vi "DevScripts_EnumToEnumAndLookup.vi"() -> ()   [LabVIEW 2024]
uses:
  <vilib>/regexp/Match Regular Expression.xnode
  SDL3/Pixels/PixelFormat--enum.ctl
  SDL3/Pixels/Pixels.lvlib
panel:
  out "Array":string[](array[string])
  out "Lookup":u32[](array[numeric]) format="%.0x"
  in  "#Define list":string="SDL_PIXELFORMAT_UNKNOWN = 0,\n    SDL_PIXELFORMAT_INDEX1LSB = 0x11100100u,\n        /* SDL_DEFINE_PIXELFORMAT(SDL_PIXELTYPE_INDEX1, SDL_BITMAPORDER_4321, 0, 1, 0), */\n    SDL_PIXELFORMAT_INDEX1MSB = 0x11200100u,\n        /* SDL_DEFINE_PIXELFORMAT(SDL_PIXELTYPE_INDEX1, SDL_BITMAPORDER_1234, 0, 1, 0), */\n    SDL_PIXELFORMAT_INDEX2LSB = 0x1c100200u,\n        /* SDL_DEFINE_PIXELFORMAT(SDL_PIXELTYPE_INDEX2, SDL_BITMAPORDER_4321, 0, 2, 0), */\n    SDL_PIXELFORMAT_INDEX2MSB = 0x1c200200u,\n        /* SDL_DEFINE_PIXELFORMAT(SDL_PIXELTYPE_INDEX2, SDL_BITMAPORDER_1234, 0, 2, 0), */\n    SDL_PIXELFORMAT_INDEX4LSB = 0x12100400u,\n        /* SDL_DEFINE_PIXELFORMAT(SDL_PIXELTYPE_INDEX4, SDL_BITMAPORDER_4321, 0, 4, 0), */\n    SDL_PIXELFORMAT_INDEX4MSB = 0x12200400u,\n        /* SDL_DEFINE_PIXELFORMAT(SDL_PIXELTYPE_INDEX4, SDL_BITMAPORDER_1234, 0, 4, 0), */\n    SDL_PIXELFORMAT_INDEX8 = 0x13000801u,\n        /* SDL_DEFINE_PIXELFORMAT(SDL_PIXELTYPE_INDEX8, 0, 0, 8, 1), */\n    SDL_PIXELFORMAT_RGB332 = 0x14110801u,\n        /* SDL_DEFINE_PIXELFORMAT(SDL_PIXELTYPE_PACKED8, SDL_PACKEDORDER_XRGB, SDL_PACKEDLAYOUT_332, 8, 1), */\n    SDL_PIXELFORMAT_XRGB4444 = 0x15120c02u,\n        /* SDL_DEFINE_PIXELFORMAT(SDL_PIXELTYPE_PACKED16, SDL_PACKEDORDER_XRGB, SDL_PACKEDLAYOUT_4444, 12, 2), */\n    SDL_PIXELFORMAT_XBGR4444 = 0x15520c02u,\n        /* SDL_DEFINE_PIXELFORMAT(SDL_PIXELTYPE_PACKED16, SDL_PACKEDORDER_XBGR, SDL_PACKEDLAYOUT_4444, 12, 2), */\n    SDL_PIXELFORMAT_XRGB1555 = 0x15130f02u,\n        /* SDL_DEFINE_PIXELFORMAT(SDL_PIXELTYPE_PACKED16, SDL_PACKEDORDER_XRGB, SDL_PACKEDLAYOUT_1555, 15, 2), */\n    SDL_PIXELFORMAT_XBGR1555 = 0x15530f02u,\n        /* SDL_DEFINE_PIXELFORMAT(SDL_PIXELTYPE_PACKED16, SDL_PACKEDORDER_XBGR, SDL_PACKEDLAYOUT_1555, 15, 2), */\n    SDL_PIXELFORMAT_ARGB4444 = 0x15321002u,\n        /* SDL_DEFINE_PIXELFORMAT(SDL_PIXELTYPE_PACKED16, SDL_PACKEDORDER_ARGB, SDL_PACKEDLAYOUT_4444, 16, 2), */\n    SDL_PIXELFORMAT_RGBA4444 = 0x15421002u,\n        /* SDL_DEFINE_PIXELFORMAT(SDL_PIXELTYPE_PACKED16, SDL_PACKEDORDER_RGBA, SDL_PACKEDLAYOUT_4444, 16, 2), */\n    SDL_PIXELFORMAT_ABGR4444 = 0x15721002u,\n        /* SDL_DEFINE_PIXELFORMAT(SDL_PIXELTYPE_PACKED16, SDL_PACKEDORDER_ABGR, SDL_PACKEDLAYOUT_4444, 16, 2), */\n    SDL_PIXELFORMAT_BGRA4444 = 0x15821002u,\n        /* SDL_DEFINE_PIXELFORMAT(SDL_PIXELTYPE_PACKED16, SDL_PACKEDORDER_BGRA, SDL_PACKEDLAYOUT_4444, 16, 2), */\n    SDL_PIXELFORMAT_ARGB1555 = 0x15331002u,\n        /* SDL_DEFINE_PIXELFORMAT(SDL_PIXELTYPE_PACKED16, SDL_PACKEDORDER_ARGB, SDL_PACKEDLAYOUT_1555, 16, 2), */\n    SDL_PIXELFORMAT_RGBA5551 = 0x15441002u,\n        /* SDL_DEFINE_PIXELFORMAT(SDL_PIXELTYPE_PACKED16, SDL_PACKEDORDER_RGBA, SDL_PACKEDLAYOUT_5551, 16, 2), */\n    SDL_PIXELFORMAT_ABGR1555 = 0x15731002u,\n        /* SDL_DEFINE_PIXELFORMAT(SDL_PIXELTYPE_PACKED16, SDL_PACKEDORDER_ABGR, SDL_PACKEDLAYOUT_1555, 16, 2), */\n    SDL_PIXELFORMAT_BGRA5551 = 0x15841002u,\n        /* SDL_DEFINE_PIXELFORMAT(SDL_PIXELTYPE_PACKED16, SDL_PACKEDORDER_BGRA, SDL_PACKEDLAYOUT_5551, 16, 2), */\n    SDL_PIXELFORMAT_RGB565 = 0x15151002u,\n        /* SDL_DEFINE_PIXELFORMAT(SDL_PIXELTYPE_PACKED16, SDL_PACKEDORDER_XRGB, SDL_PACKEDLAYOUT_565, 16, 2), */\n    SDL_PIXELFORMAT_BGR565 = 0x15551002u,\n        /* SDL_DEFINE_PIXELFORMAT(SDL_PIXELTYPE_PACKED16, SDL_PACKEDORDER_XBGR, SDL_PACKEDLAYOUT_565, 16, 2), */\n    SDL_PIXELFORMAT_RGB24 = 0x17101803u,\n        /* SDL_DEFINE_PIXELFORMAT(SDL_PIXELTYPE_ARRAYU8, SDL_ARRAYORDER_RGB, 0, 24, 3), */\n    SDL_PIXELFORMAT_BGR24 = 0x17401803u,\n        /* SDL_DEFINE_PIXELFORMAT(SDL_PIXELTYPE_ARRAYU8, SDL_ARRAYORDER_BGR, 0, 24, 3), */\n    SDL_PIXELFORMAT_XRGB8888 = 0x16161804u,\n        /* SDL_DEFINE_PIXELFORMAT(SDL_PIXELTYPE_PACKED32, SDL_PACKEDORDER_XRGB, SDL_PACKEDLAYOUT_8888, 24, 4), */\n    SDL_PIXELFORMAT_RGBX8888 = 0x16261804u,\n        /* SDL_DEFINE_PIXELFORMAT(SDL_PIXELTYPE_PACKED32, SDL_PACKEDORDER_RGBX, SDL_PACKEDLAYOUT_8888, 24, 4), */\n    SDL_PIXELFORMAT_XBGR8888 = 0x16561804u,\n        /* SDL_DEFINE_PIXELFORMAT(SDL_PIXELTYPE_PACKED32, SDL_PACKEDORDER_XBGR, SDL_PACKEDLAYOUT_8888, 24, 4), */\n    SDL_PIXELFORMAT_BGRX8888 = 0x16661804u,\n        /* SDL_DEFINE_PIXELFORMAT(SDL_PIXELTYPE_PACKED32, SDL_PACKEDORDER_BGRX, SDL_PACKEDLAYOUT_8888, 24, 4), */\n    SDL_PIXELFORMAT_ARGB8888 = 0x16362004u,\n        /* SDL_DEFINE_PIXELFORMAT(SDL_PIXELTYPE_PACKED32, SDL_PACKEDORDER_ARGB, SDL_PACKEDLAYOUT_8888, 32, 4), */\n    SDL_PIXELFORMAT_RGBA8888 = 0x16462004u,\n        /* SDL_DEFINE_PIXELFORMAT(SDL_PIXELTYPE_PACKED32, SDL_PACKEDORDER_RGBA, SDL_PACKEDLAYOUT_8888, 32, 4), */\n    SDL_PIXELFORMAT_ABGR8888 = 0x16762004u,\n        /* SDL_DEFINE_PIXELFORMAT(SDL_PIXELTYPE_PACKED32, SDL_PACKEDORDER_ABGR, SDL_PACKEDLAYOUT_8888, 32, 4), */\n    SDL_PIXELFORMAT_BGRA8888 = 0x16862004u,\n        /* SDL_DEFINE_PIXELFORMAT(SDL_PIXELTYPE_PACKED32, SDL_PACKEDORDER_BGRA, SDL_PACKEDLAYOUT_8888, 32, 4), */\n    SDL_PIXELFORMAT_XRGB2101010 = 0x16172004u,\n        /* SDL_DEFINE_PIXELFORMAT(SDL_PIXELTYPE_PACKED32, SDL_PACKEDORDER_XRGB, SDL_PACKEDLAYOUT_2101010, 32, 4), */\n    SDL_PIXELFORMAT_XBGR2101010 = 0x16572004u,\n        /* SDL_DEFINE_PIXELFORMAT(SDL_PIXELTYPE_PACKED32, SDL_PACKEDORDER_XBGR, SDL_PACKEDLAYOUT_2101010, 32, 4), */\n    SDL_PIXELFORMAT_ARGB2101010 = 0x16372004u,\n        /* SDL_DEFINE_PIXELFORMAT(SDL_PIXELTYPE_PACKED32, SDL_PACKEDORDER_ARGB, SDL_PACKEDLAYOUT_2101010, 32, 4), */\n    SDL_PIXELFORMAT_ABGR2101010 = 0x16772004u,\n        /* SDL_DEFINE_PIXELFORMAT(SDL_PIXELTYPE_PACKED32, SDL_PACKEDORDER_ABGR, SDL_PACKEDLAYOUT_2101010, 32, 4), */\n    SDL_PIXELFORMAT_RGB48 = 0x18103006u,\n        /* SDL_DEFINE_PIXELFORMAT(SDL_PIXELTYPE_ARRAYU16, SDL_ARRAYORDER_RGB, 0, 48, 6), */\n    SDL_PIXELFORMAT_BGR48 = 0x18403006u,\n        /* SDL_DEFINE_PIXELFORMAT(SDL_PIXELTYPE_ARRAYU16, SDL_ARRAYORDER_BGR, 0, 48, 6), */\n    SDL_PIXELFORMAT_RGBA64 = 0x18204008u,\n        /* SDL_DEFINE_PIXELFORMAT(SDL_PIXELTYPE_ARRAYU16, SDL_ARRAYORDER_RGBA, 0, 64, 8), */\n    SDL_PIXELFORMAT_ARGB64 = 0x18304008u,\n        /* SDL_DEFINE_PIXELFORMAT(SDL_PIXELTYPE_ARRAYU16, SDL_ARRAYORDER_ARGB, 0, 64, 8), */\n    SDL_PIXELFORMAT_BGRA64 = 0x18504008u,\n        /* SDL_DEFINE_PIXELFORMAT(SDL_PIXELTYPE_ARRAYU16, SDL_ARRAYORDER_BGRA, 0, 64, 8), */\n    SDL_PIXELFORMAT_ABGR64 = 0x18604008u,\n        /* SDL_DEFINE_PIXELFORMAT(SDL_PIXELTYPE_ARRAYU16, SDL_ARRAYORDER_ABGR, 0, 64, 8), */\n    SDL_PIXELFORMAT_RGB48_FLOAT = 0x1a103006u,\n        /* SDL_DEFINE_PIXELFORMAT(SDL_PIXELTYPE_ARRAYF16, SDL_ARRAYORDER_RGB, 0, 48, 6), */\n    SDL_PIXELFORMAT_BGR48_FLOAT = 0x1a403006u,\n        /* SDL_DEFINE_PIXELFORMAT(SDL_PIXELTYPE_ARRAYF16, SDL_ARRAYORDER_BGR, 0, 48, 6), */\n    SDL_PIXELFORMAT_RGBA64_FLOAT = 0x1a204008u,\n        /* SDL_DEFINE_PIXELFORMAT(SDL_PIXELTYPE_ARRAYF16, SDL_ARRAYORDER_RGBA, 0, 64, 8), */\n    SDL_PIXELFORMAT_ARGB64_FLOAT = 0x1a304008u,\n        /* SDL_DEFINE_PIXELFORMAT(SDL_PIXELTYPE_ARRAYF16, SDL_ARRAYORDER_ARGB, 0, 64, 8), */\n    SDL_PIXELFORMAT_BGRA64_FLOAT = 0x1a504008u,\n        /* SDL_DEFINE_PIXELFORMAT(SDL_PIXELTYPE_ARRAYF16, SDL_ARRAYORDER_BGRA, 0, 64, 8), */\n    SDL_PIXELFORMAT_ABGR64_FLOAT = 0x1a604008u,\n        /* SDL_DEFINE_PIXELFORMAT(SDL_PIXELTYPE_ARRAYF16, SDL_ARRAYORDER_ABGR, 0, 64, 8), */\n    SDL_PIXELFORMAT_RGB96_FLOAT = 0x1b10600cu,\n        /* SDL_DEFINE_PIXELFORMAT(SDL_PIXELTYPE_ARRAYF32, SDL_ARRAYORDER_RGB, 0, 96, 12), */\n    SDL_PIXELFORMAT_BGR96_FLOAT = 0x1b40600cu,\n        /* SDL_DEFINE_PIXELFORMAT(SDL_PIXELTYPE_ARRAYF32, SDL_ARRAYORDER_BGR, 0, 96, 12), */\n    SDL_PIXELFORMAT_RGBA128_FLOAT = 0x1b208010u,\n        /* SDL_DEFINE_PIXELFORMAT(SDL_PIXELTYPE_ARRAYF32, SDL_ARRAYORDER_RGBA, 0, 128, 16), */\n    SDL_PIXELFORMAT_ARGB128_FLOAT = 0x1b308010u,\n        /* SDL_DEFINE_PIXELFORMAT(SDL_PIXELTYPE_ARRAYF32, SDL_ARRAYORDER_ARGB, 0, 128, 16), */\n    SDL_PIXELFORMAT_BGRA128_FLOAT = 0x1b508010u,\n        /* SDL_DEFINE_PIXELFORMAT(SDL_PIXELTYPE_ARRAYF32, SDL_ARRAYORDER_BGRA, 0, 128, 16), */\n    SDL_PIXELFORMAT_ABGR128_FLOAT = 0x1b608010u,\n        /* SDL_DEFINE_PIXELFORMAT(SDL_PIXELTYPE_ARRAYF32, SDL_ARRAYORDER_ABGR, 0, 128, 16), */\n    SDL_PIXELFORMAT_YV12 = 0x32315659u,      \n/**< Planar mode: Y + V + U  (3 planes) */\n        /* SDL_DEFINE_PIXELFOURCC('Y', 'V', '1', '2'), */\n    SDL_PIXELFORMAT_IYUV = 0x56555949u,      \n/**< Planar mode: Y + U + V  (3 planes) */\n        /* SDL_DEFINE_PIXELFOURCC('I', 'Y', 'U', 'V'), */\n    SDL_PIXELFORMAT_YUY2 = 0x32595559u,      \n/**< Packed mode: Y0+U0+Y1+V0 (1 plane) */\n        /* SDL_DEFINE_PIXELFOURCC('Y', 'U', 'Y', '2'), */\n    SDL_PIXELFORMAT_UYVY = 0x59565955u,      \n/**< Packed mode: U0+Y0+V0+Y1 (1 plane) */\n        /* SDL_DEFINE_PIXELFOURCC('U', 'Y', 'V', 'Y'), */\n    SDL_PIXELFORMAT_YVYU = 0x55595659u,      \n/**< Packed mode: Y0+V0+Y1+U0 (1 plane) */\n        /* SDL_DEFINE_PIXELFOURCC('Y', 'V', 'Y', 'U'), */\n    SDL_PIXELFORMAT_NV12 = 0x3231564eu,     \n/**< Planar mode: Y + U/V interleaved  (2 planes) */\n        /* SDL_DEFINE_PIXELFOURCC('N', 'V', '1', '2'), */\n    SDL_PIXELFORMAT_NV21 = 0x3132564eu,     \n/**< Planar mode: Y + V/U interleaved  (2 planes) */\n        /* SDL_DEFINE_PIXELFOURCC('N', 'V', '2', '1'), */\n    SDL_PIXELFORMAT_P010 = 0x30313050u,     \n/**< Planar mode: Y + U/V interleaved  (2 planes) */\n        /* SDL_DEFINE_PIXELFOURCC('P', '0', '1', '0'), */\n    SDL_PIXELFORMAT_EXTERNAL_OES = 0x2053454fu,   \n  /**< Android video texture format */\n        /* SDL_DEFINE_PIXELFOURCC('O', 'E', 'S', ' ') */"
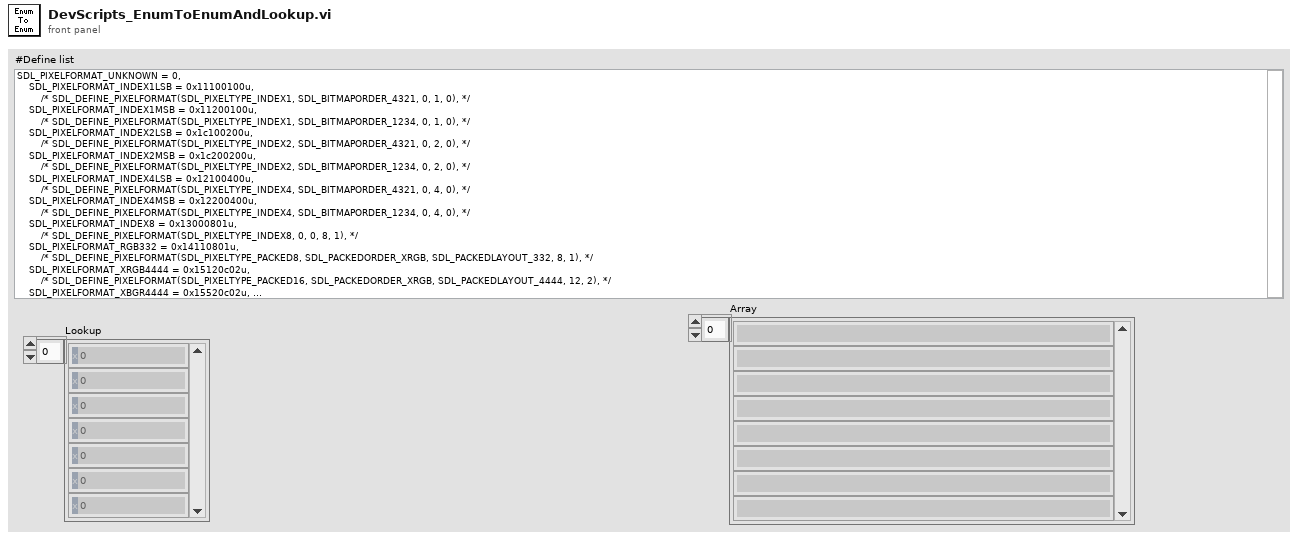
[diagram p1: front panel]
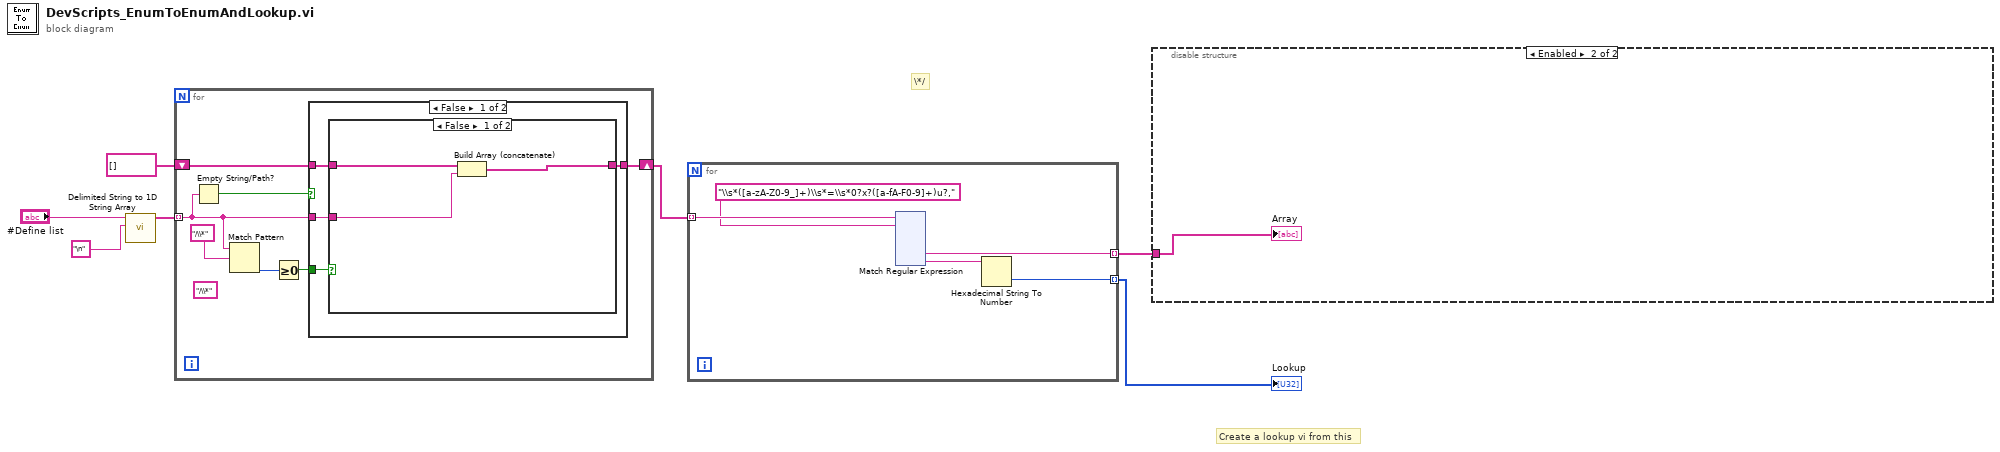
[diagram p0: block diagram]
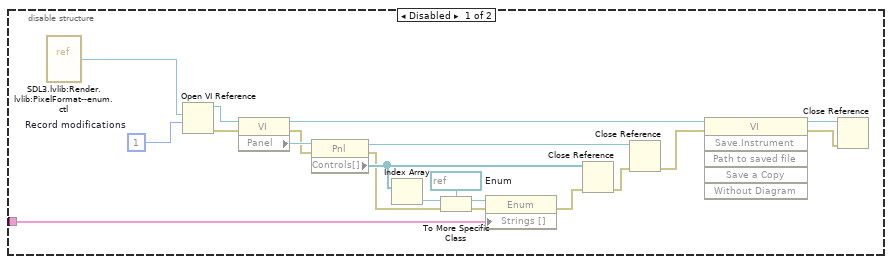
[diagram p2: hidden frame]
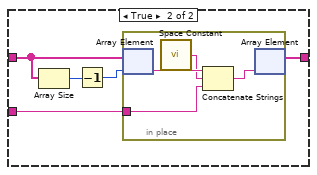
[diagram p3: hidden frame]
diagram:
  # "Create a lookup vi from this"
  # "\\*/"
  n1 = call <vilib>:"Delimited String to 1D String Array.vi"("delimiter"="\n", "delimited string"="#Define list") -> ("string array"=w5:string[])  [unwired: 9 in]
  n2 = for {
    tunnel: w5 -> [w9] mode=indexing
    shift-right: [w12] -> w3
    shift-left: string[] [] -> [w13]
    (unwired) "/\\*" ("regular expression")
    n3 = Empty String/Path?(string/path=w9) -> (empty?=w8:bool)
    n4 = Match Pattern(string=w9, regular expression="/\\*") -> (offset past match=w11:i32)  [unwired: 1 in, 3 out]
    n5 = Greater Or Equal To 0?(x=w11) -> (x >= 0?=w10:bool)
    n6 = case shown="False" w8 {
      tunnel: w13 -> [w18 w31]
      tunnel: [w17 w31] -> w12
      tunnel: w10 -> [w16 _]
      tunnel: w9 -> [w15 _]
      frame False {
        n7 = case shown="False" w16 {
          tunnel: w18 -> [w21 w26]
          tunnel: [w20 w25] -> w17
          tunnel: w15 -> [w19 w24]
          frame False {
            n8 = Build Array (concatenate)(w21, w19) -> (w20:string[])
          }
          frame True {
            n9 = Array Size(array=w26) -> (size(s)=w23:i32)
            n10 = Decrement(x=w23) -> (x-1=w22:i32)
            n11 = in-place {
              in-place-border: w24 -> [w27]
              n12 = in-place-array #1(w26, w22) -> (w30:string)
              n13 = call <vilib>:"Space Constant.vi"() -> ("String"=w28:string)
              n14 = Concatenate Strings(w30, w28, w27) -> (w29:string)
              n15 = in-place-array #1(w29) -> (w25:string[])  [unwired: 1 out]
            }
          }
        }
      }
      frame True {
      }
    }
  }
  n16 = for {
    tunnel: w3 -> [w36] mode=indexing
    tunnel: [w33] -> w1 mode=indexing
    tunnel: [w32] -> w2 mode=indexing
    n17 = xnode "Match Regular Expression"("input string"=w36, "regular expression"="\\s*([a-zA-Z0-9_]+)\\s*=\\s*0?x?([a-fA-F0-9]+)u?,") -> ("submatch 1"=w32:string, "submatch 2"=w34:string)  [unwired: 4 in, 5 out]
    n18 = Hexadecimal String To Number(string=w34) -> (number=w33:u32)  [unwired: 2 in, 1 out]
  }
  "Lookup" <- w1
  n19 = disable-structure shown="Enabled" {
    disable-tunnel: w2 -> [w158 w177]
    frame Disabled {
      w168 = refnum<vi> refnum  # Enum
      w174 = 1  # Record modifications
      n20 = vi-ref "SDL3.lvlib:Render.lvlib:PixelFormat--enum.ctl"() -> (w175:refnum<vi>)
      n21 = Open VI Reference(vi path=w175, options=w174) -> (vi reference=w173:refnum<vi>, error out=w176:errorcluster)  [unwired: 4 in]
      n22 = property class="VI"(reference=w173, error in=w176) -> (reference out=w163:refnum<vi>, error out=w171:errorcluster, "Panel"=w172:refnum<vi>)
      n23 = property class="Pnl"(reference=w172, error in=w171) -> (reference out=w170:refnum<vi>, error out=w161:errorcluster, "Controls[]"=w166:refnum<vi>[])
      n24 = Index Array(array=w166) -> (element=w167:refnum<vi>)  [unwired: 1 in]
      n25 = To More Specific Class(target class=w168, reference=w167, error in=w161) -> (specific class reference=w160:refnum<vi>, error out=w159:errorcluster)
      n26 = property class="Enum"(reference=w160, error in=w159, "Strings []"=w158) -> (error out=w157:errorcluster)  [unwired: 1 out]
      n27 = Close Reference(reference=w166, error in (no error)=w157) -> (error out=w165:errorcluster)
      n28 = Close Reference(reference=w170, error in (no error)=w165) -> (error out=w169:errorcluster)
      n29 = invoke class="VI" method="Save.Instrument"(reference=w163, error in=w169) -> (reference out=w162:refnum<vi>, error out=w164:errorcluster)  [unwired: 4 in, 4 out]
      n30 = Close Reference(reference=w162, error in (no error)=w164) -> ()  [unwired: 1 out]
    }
    frame Enabled {
      "Array" <- w177
    }
  }
